vi "CVT MUS2MIDI controller.vi"(8 "error in":errorcluster, 11 "MSU set":u8) -> (0 "error out":errorcluster, 3 "midi_ctrl":u8)   [LabVIEW 2014]
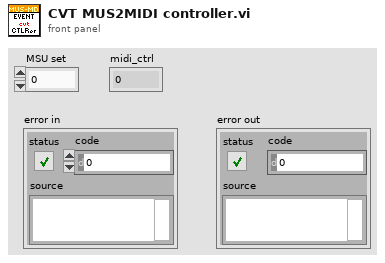
[diagram p1: front panel]
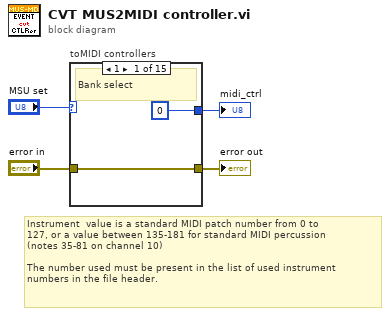
[diagram p0: block diagram]
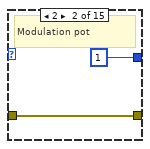
[diagram p2: hidden frame]
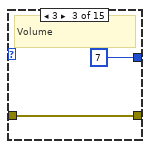
[diagram p3: hidden frame]
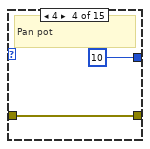
[diagram p4: hidden frame]
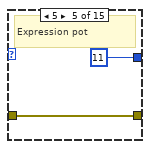
[diagram p5: hidden frame]
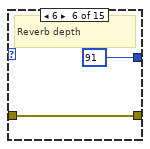
[diagram p6: hidden frame]
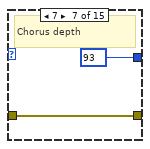
[diagram p7: hidden frame]
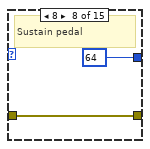
[diagram p8: hidden frame]
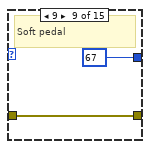
[diagram p9: hidden frame]
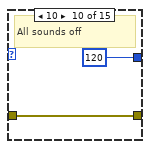
[diagram p10: hidden frame]
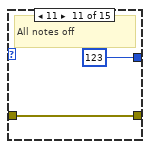
[diagram p11: hidden frame]
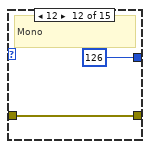
[diagram p12: hidden frame]
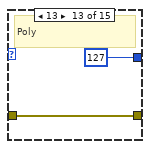
[diagram p13: hidden frame]
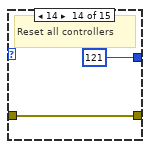
[diagram p14: hidden frame]
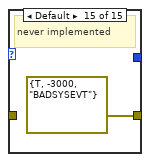
[diagram p15: hidden frame]
diagram:
  # "Instrument  value is a standard MIDI patch number from 0 to \n127, or a value between 135-181 for standard MIDI percussion \n(notes 35-81 on channel 10)\n\nThe number used must be present in the list of used instrument \nnumbers in the file header."
  n1 = case "toMIDI controllers" shown="1" "MSU set" {
    tunnel: [u8 0 ("data") u8 1 ("data") u8 7 ("data") u8 10 ("data") u8 11 ("data") u8 91 ("data") u8 93 ("data") u8 64 ("data") u8 67 ("data") u8 120 ("data") u8 123 ("data") u8 126 ("data") u8 127 ("data") u8 121 ("data") _] -> w2
    tunnel: [w5 w7 w9 w11 w13 w15 w17 w19 w21 w23 w25 w27 w29 w31 errorcluster {"status"=TRUE, "code"=-3000, "source"="BADSYSEVT"} ("error constant")] -> w4
    tunnel: "error in" -> [w5 w7 w9 w11 w13 w15 w17 w19 w21 w23 w25 w27 w29 w31 _]
    frame 1 {
      # "Bank select"
    }
    frame 2 {
      # "Modulation pot"
    }
    frame 3 {
      # "Volume"
    }
    frame 4 {
      # "Pan pot"
    }
    frame 5 {
      # "Expression pot"
    }
    frame 6 {
      # "Reverb depth"
    }
    frame 7 {
      # "Chorus depth"
    }
    frame 8 {
      # "Sustain pedal"
    }
    frame 9 {
      # "Soft pedal"
    }
    frame 10 {
      # "All sounds off"
    }
    frame 11 {
      # "All notes off"
    }
    frame 12 {
      # "Mono"
    }
    frame 13 {
      # "Poly"
    }
    frame 14 {
      # "Reset all controllers"
    }
    frame Default {
      # "never implemented"
    }
  }
  "error out" <- w4
  "midi_ctrl" <- w2
